vi "File Example.vi"() -> ()   [LabVIEW 2020]
uses:
  Source/Type Defs/Debug Level.ctl
  Source/LV Log.lvlib
  Source/Logger/Logger.lvclass
panel:
  in  "Log Path":path
  in  "error in (no error)":errorcluster
  in  "Debug Level":T1=enum."DEBUG"
  out "error out":errorcluster
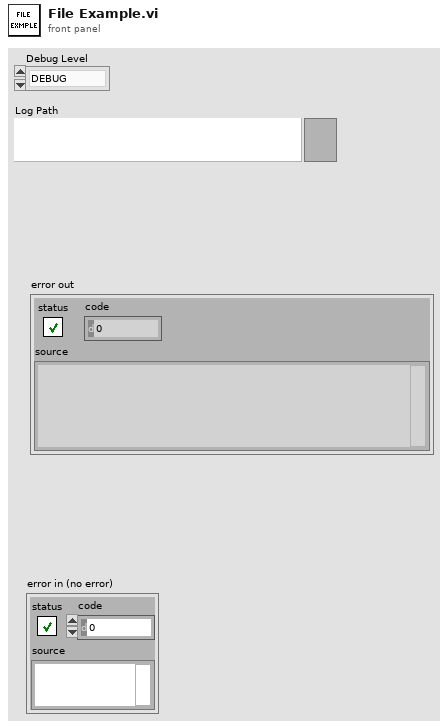
[diagram p1: front panel]
types:
  T1 = typedef "LV Log.lvlib/Debug Level.ctl" = enum16{"DEFAULT", "DEBUG", "INFO", "WARN", "ERROR", "FATAL"}
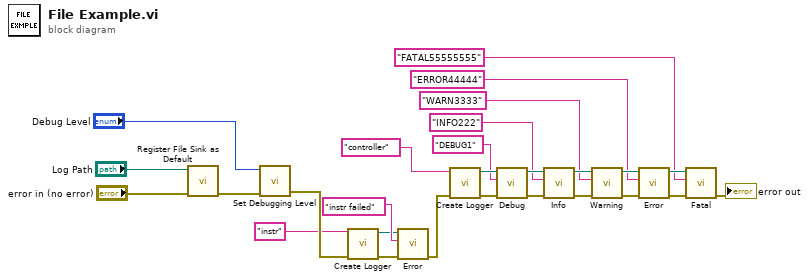
[diagram p0: block diagram]
diagram:
  n1 = call "Register File Sink as Default.vi"("error in (no error)"="error in (no error)", "Path"="Log Path") -> ("error out"=w26:errorcluster)  [unwired: 9 in]
  n2 = call "Set Debugging Level.vi"("error in (no error)"=w26, "Debug Level in"="Debug Level") -> ("error out"=w4:errorcluster)  [unwired: 9 in]
  n3 = call "Create Logger.vi"("error in (no error)"=w4, "Name"="instr") -> ("error out"=w2:errorcluster, "Logger out"=w3:refnum<class "Logger.lvclass">)  [unwired: 8 in]
  n4 = call "Error.vi"("error in (no error)"=w2, "Log Text"="instr failed", "Logger in"=w3) -> ("error out"=w5:errorcluster)  [unwired: 6 in, 2 out]
  n5 = call "Create Logger.vi"("error in (no error)"=w5, "Name"="controller") -> ("error out"=w24:errorcluster, "Logger out"=w23:refnum<class "Logger.lvclass">)  [unwired: 8 in]
  n6 = call "Debug.vi"("error in (no error)"=w24, "Log Text"="DEBUG1", "Logger in"=w23) -> ("error out"=w21:errorcluster, "Logger out"=w22:refnum<class "Logger.lvclass">)  [unwired: 6 in, 1 out]
  n7 = call "Info.vi"("error in (no error)"=w21, "Log Text"="INFO222", "Logger in"=w22) -> ("error out"=w20:errorcluster, "Logger out"=w19:refnum<class "Logger.lvclass">)  [unwired: 6 in, 1 out]
  n8 = call "Warning.vi"("error in (no error)"=w20, "Log Text"="WARN3333", "Logger in"=w19) -> ("error out"=w17:errorcluster, "Logger out"=w18:refnum<class "Logger.lvclass">)  [unwired: 6 in, 1 out]
  n9 = call "Error.vi"("error in (no error)"=w17, "Log Text"="ERROR44444", "Logger in"=w18) -> ("error out"=w16:errorcluster, "Logger out"=w15:refnum<class "Logger.lvclass">)  [unwired: 6 in, 1 out]
  n10 = call "Fatal.vi"("error in (no error)"=w16, "Log Text"="FATAL55555555", "Logger in"=w15) -> ("error out"=→"error out":errorcluster)  [unwired: 6 in, 2 out]
